vi "CMC_Homework_03_V2.vi"() -> ()   [LabVIEW 2013]
uses:
  <vilib>/gmath/NI_Gmath.lvlib
panel:
  in  "Formulae":string="x*ln(x)*sin(x^2)"
  in  "stop":bool
  out "Middle Bound":dbl
  in  "Lower Bound":dbl
  in  "Upper Bound":dbl
  in  "Tolerance":dbl min=0.0
  out "Calculated Tolerance":dbl
  out "Roots of F(x) found to Tolerance":string[](array[string])
  # "Created in Collaboration with Sarah Bailey & Alex Offredi"
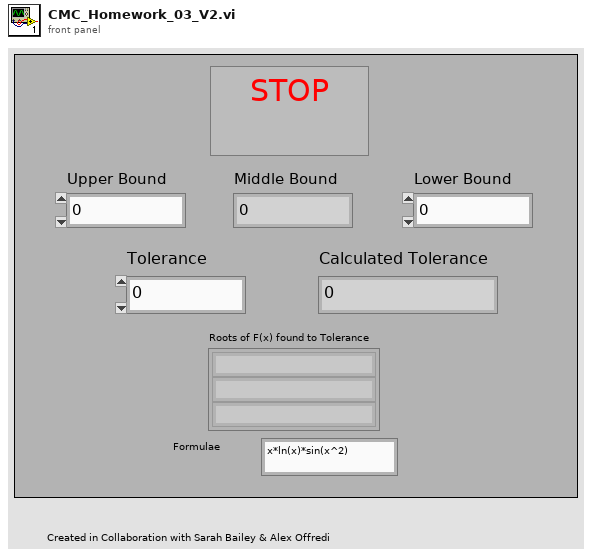
[diagram p1: front panel]
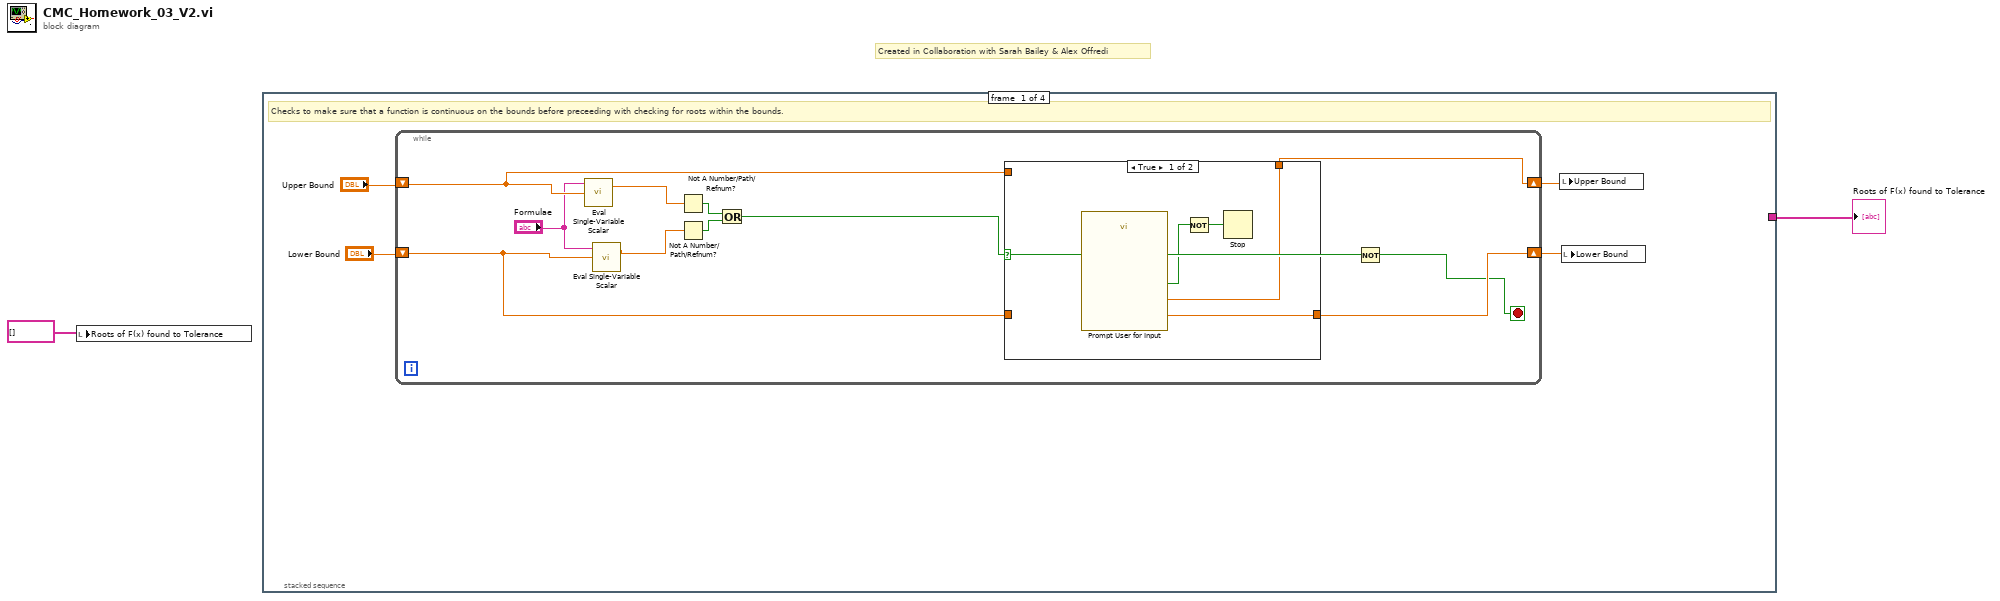
[diagram p0: block diagram]
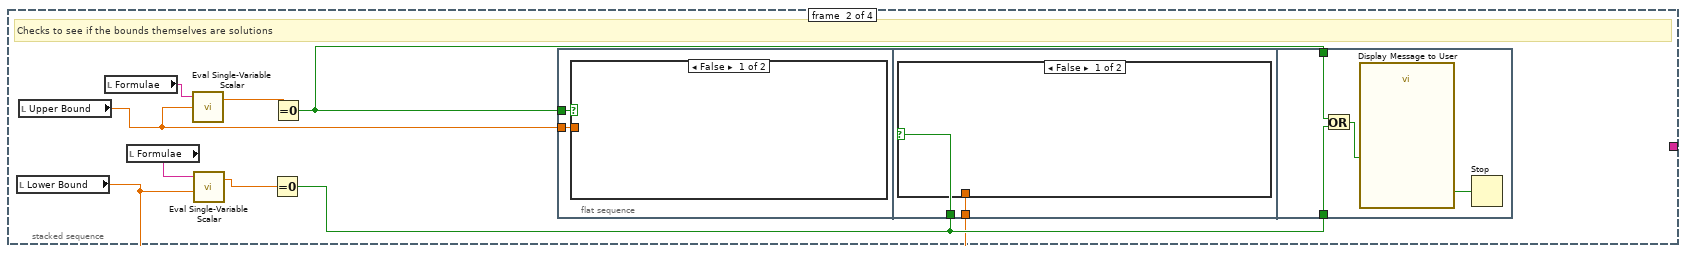
[diagram p3: hidden frame]
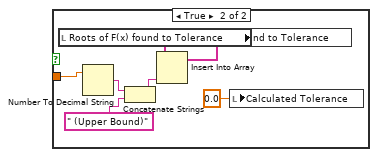
[diagram p4: hidden frame]
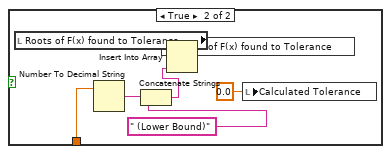
[diagram p5: hidden frame]
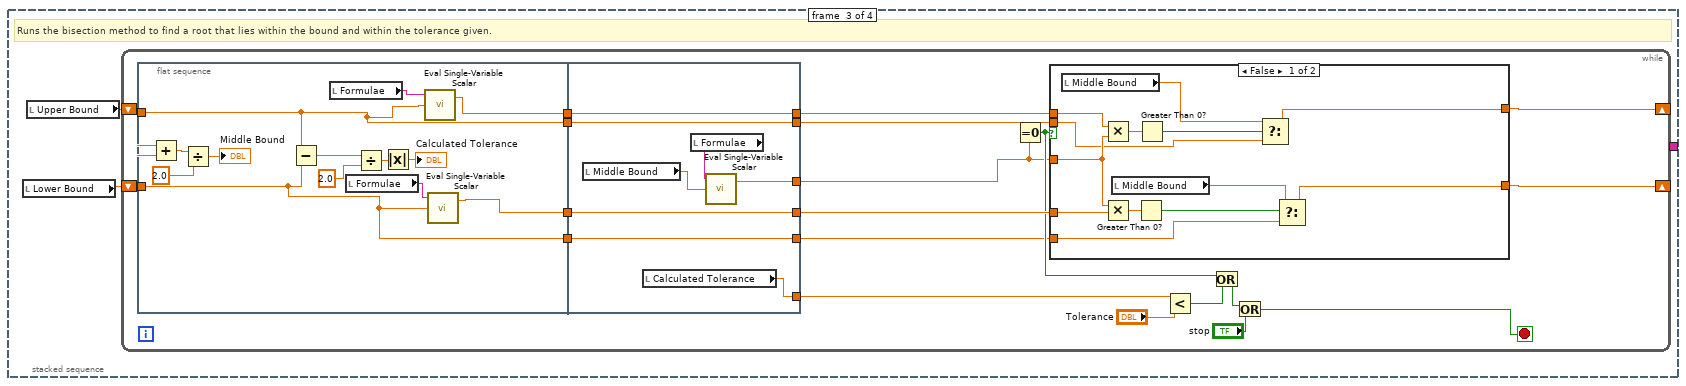
[diagram p6: hidden frame]
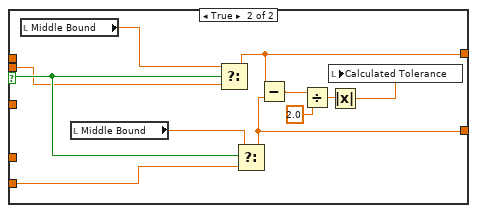
[diagram p7: hidden frame]
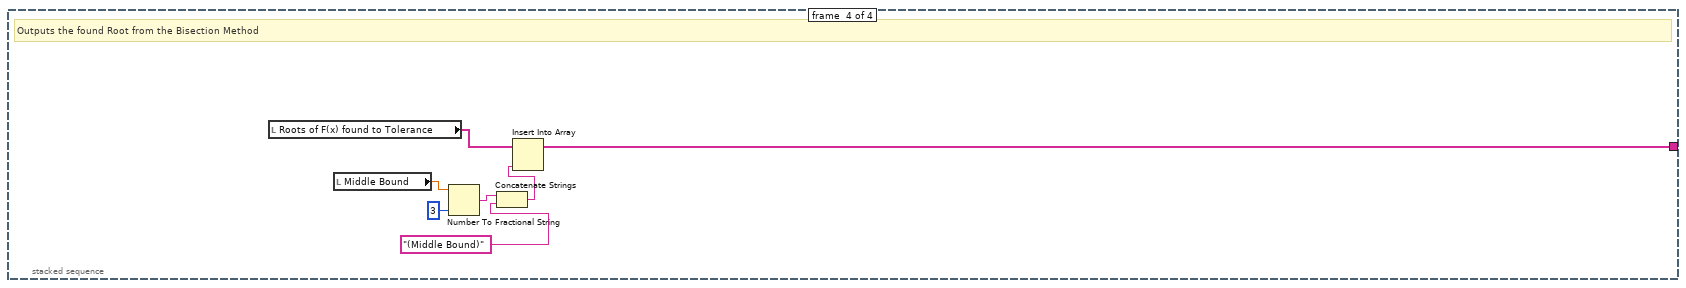
[diagram p8: hidden frame]
diagram:
  # "Created in Collaboration with Sarah Bailey & Alex Offredi"
  n1 = local write "Roots of F(x) found to Tolerance"(string[] [] ("Roots of F(x) found to Tolerance")) -> ()
  n2 = stacked-sequence {
    tunnel: [_ _ _ w122] -> w2
    frame #0 {
      # "Checks to make sure that a function is continuous on the bounds before preceeding with checking for roots within the bounds."
      n3 = while {
        shift-right: [w15] -> w3
        shift-left: "Upper Bound" -> [w11]
        shift-right: [w14] -> w4
        shift-left: "Lower Bound" -> [w9]
        stop <- w12 stop-if-true
        n4 = call <vilib>:"Eval Single-Variable Scalar.vi"("x value"=w11, "formula"="Formulae") -> ("y value"=w7:dbl)  [unwired: 1 in, 1 out]
        n5 = call <vilib>:"Eval Single-Variable Scalar.vi"("x value"=w9, "formula"="Formulae") -> ("y value"=w8:dbl)  [unwired: 1 in, 1 out]
        n6 = Not A Number/Path/Refnum?(number/path/refnum=w7) -> (NaN/Path/Refnum?=w16:bool)
        n7 = Not A Number/Path/Refnum?(number/path/refnum=w8) -> (NaN/Path/Refnum?=w17:bool)
        n8 = Or(x=w16, y=w17) -> (x .or. y?=w13:bool)
        n9 = case shown="True" w13 {
          tunnel: [w19 w22] -> w15
          tunnel: [w18 w23] -> w14
          tunnel: w11 -> [_ w22]
          tunnel: w9 -> [_ w23]
          frame True {
            n10 = call "Prompt User for Input"() -> ("Lower Bound"=w18:dbl, "Upper Bound"=w19:dbl, "OK"=w20:bool)  [unwired: 16 in, 1 out]
            n11 = Not(x=w20) -> (.not. x?=w21:bool)
            n12 = Stop(stop? (T)=w21) -> ()
          }
          frame False {
          }
        }
        n13 = Not(x=w13) -> (.not. x?=w12:bool)
      }
      n14 = local write "Upper Bound"(w3) -> ()
      n15 = local write "Lower Bound"(w4) -> ()
    }
    frame #1 {
      # "Checks to see if the bounds themselves are solutions"
      n16 = local read "Lower Bound"() -> (w25:dbl)
      n17 = local read "Upper Bound"() -> (w28:dbl)
      n18 = local read "Formulae"() -> (w29:string)
      n19 = local read "Formulae"() -> (w26:string)
      n20 = call <vilib>:"Eval Single-Variable Scalar.vi"("x value"=w28, "formula"=w29) -> ("y value"=w27:dbl)  [unwired: 1 in, 1 out]
      n21 = call <vilib>:"Eval Single-Variable Scalar.vi"("x value"=w25, "formula"=w26) -> ("y value"=w24:dbl)  [unwired: 1 in, 1 out]
      n22 = Equal To 0?(x=w24) -> (x = 0?=w31:bool)
      n23 = Equal To 0?(x=w27) -> (x = 0?=w30:bool)
      n24 = flat-sequence {
        tunnel: w30 -> [w33]
        tunnel: w28 -> [w32]
        tunnel: w31 -> [w41]
        tunnel: w25 -> [w42]
        tunnel: w31 -> [w52]
        tunnel: w30 -> [w53]
        frame #0 {
          n25 = case shown="False" w33 {
            tunnel: w32 -> [_ w38]
            frame False {
            }
            frame True {
              n26 = local read "Roots of F(x) found to Tolerance"() -> (w40:string[])
              n27 = Number To Decimal String(number=w38) -> (decimal integer string=w37:string)  [unwired: 1 in]
              n28 = Concatenate Strings(w37, " (Upper Bound)") -> (w35:string)
              n29 = Insert Into Array(array=w40, new element=w35) -> (w39:string[])  [unwired: 1 in]
              n30 = local write "Roots of F(x) found to Tolerance"(w39) -> ()
              n31 = local write "Calculated Tolerance"(0.0 ("Calculated Tolerance")) -> ()
            }
          }
        }
        frame #1 {
          n32 = case shown="False" w41 {
            tunnel: w42 -> [_ w47]
            frame False {
            }
            frame True {
              n33 = local read "Roots of F(x) found to Tolerance"() -> (w49:string[])
              n34 = Number To Decimal String(number=w47) -> (decimal integer string=w46:string)  [unwired: 1 in]
              n35 = Concatenate Strings(w46, " (Lower Bound)") -> (w44:string)
              n36 = Insert Into Array(array=w49, new element=w44) -> (w48:string[])  [unwired: 1 in]
              n37 = local write "Roots of F(x) found to Tolerance"(w48) -> ()
              n38 = local write "Calculated Tolerance"(0.0 ("Calculated Tolerance")) -> ()
            }
          }
        }
        frame #2 {
          n39 = Or(x=w53, y=w52) -> (x .or. y?=w51:bool)
          n40 = call "Display Message to User"("Enable"=w51) -> ("OK"=w50:bool)  [unwired: 9 in, 1 out]
          n41 = Stop(stop? (T)=w50) -> ()
        }
      }
    }
    frame #2 {
      # "Runs the bisection method to find a root that lies within the bound and within the tolerance given."
      n42 = local read "Lower Bound"() -> (w54:dbl)
      n43 = local read "Upper Bound"() -> (w55:dbl)
      n44 = while {
        shift-right: [w71] -> _
        shift-left: w55 -> [w75]
        shift-right: [w70] -> _
        shift-left: w54 -> [w74]
        stop <- w68 stop-if-true
        n45 = flat-sequence {
          tunnel: w75 -> [w105]
          tunnel: w74 -> [w102]
          tunnel: [w104] -> w61
          tunnel: [w103] -> w60
          tunnel: [w105] -> w59
          tunnel: [w102] -> w58
          tunnel: [w117] -> w62
          tunnel: [w118] -> w63
          tunnel: [w119] -> w72
          tunnel: [w120] -> w73
          tunnel: w61 -> [w120]
          tunnel: w60 -> [w119]
          tunnel: w59 -> [w118]
          tunnel: w58 -> [w117]
          tunnel: [w114] -> w57
          tunnel: [w113] -> w56
          frame #0 {
            n46 = Add(x=w105, y=w102) -> (x+y=w111:dbl)
            n47 = Divide(x=w111, y=2.0) -> (x/y=→"Middle Bound":dbl)
            n48 = Subtract(x=w105, y=w102) -> (x-y=w109:dbl)
            n49 = local read "Formulae"() -> (w101:string)
            n50 = local read "Formulae"() -> (w100:string)
            n51 = Divide(x=w109, y=2.0) -> (x/y=w107:dbl)
            n52 = Absolute Value(x=w107) -> (abs(x)=→"Calculated Tolerance":dbl)
            n53 = call <vilib>:"Eval Single-Variable Scalar.vi"("x value"=w105, "formula"=w101) -> ("y value"=w104:dbl)  [unwired: 1 in, 1 out]
            n54 = call <vilib>:"Eval Single-Variable Scalar.vi"("x value"=w102, "formula"=w100) -> ("y value"=w103:dbl)  [unwired: 1 in, 1 out]
          }
          frame #1 {
            n55 = local read "Middle Bound"() -> (w116:dbl)
            n56 = local read "Calculated Tolerance"() -> (w113:dbl)
            n57 = local read "Formulae"() -> (w115:string)
            n58 = call <vilib>:"Eval Single-Variable Scalar.vi"("x value"=w116, "formula"=w115) -> ("y value"=w114:dbl)  [unwired: 1 in, 1 out]
          }
        }
        n59 = Equal To 0?(x=w57) -> (x = 0?=w66:bool)
        n60 = case shown="False" w66 {
          selector: w66 -> [_ w91]
          tunnel: w73 -> [w78 _]
          tunnel: w72 -> [w80 _]
          tunnel: [w85 w95] -> w71
          tunnel: w57 -> [w79 _]
          tunnel: [w82 w94] -> w70
          tunnel: w63 -> [w77 w89]
          tunnel: w62 -> [w76 w90]
          frame False {
            n61 = local read "Middle Bound"() -> (w81:dbl)
            n62 = Multiply(x=w78, y=w79) -> (x*y=w88:dbl)
            n63 = Multiply(x=w79, y=w80) -> (x*y=w87:dbl)
            n64 = local read "Middle Bound"() -> (w83:dbl)
            n65 = Greater Than 0?(x=w87) -> (x > 0?=w84:bool)
            n66 = Greater Than 0?(x=w88) -> (x > 0?=w86:bool)
            n67 = Select(t=w81, s=w86, f=w77) -> (s? t:f=w85:dbl)
            n68 = Select(t=w83, s=w84, f=w76) -> (s? t:f=w82:dbl)
          }
          frame True {
            n69 = local read "Middle Bound"() -> (w98:dbl)
            n70 = local read "Middle Bound"() -> (w99:dbl)
            n71 = Select(t=w98, s=w91, f=w89) -> (s? t:f=w95:dbl)
            n72 = Select(t=w99, s=w91, f=w90) -> (s? t:f=w94:dbl)
            n73 = Subtract(x=w95, y=w94) -> (x-y=w96:dbl)
            n74 = Divide(x=w96, y=2.0) -> (x/y=w93:dbl)
            n75 = Absolute Value(x=w93) -> (abs(x)=w92:dbl)
            n76 = local write "Calculated Tolerance"(w92) -> ()
          }
        }
        n77 = Less?(x=w56, y="Tolerance") -> (x < y?=w65:bool)
        n78 = Or(x=w66, y=w65) -> (x .or. y?=w64:bool)
        n79 = Or(x=w64, y="stop") -> (x .or. y?=w68:bool)
      }
    }
    frame #3 {
      # "Outputs the found Root from the Bisection Method"
      n80 = local read "Roots of F(x) found to Tolerance"() -> (w127:string[])
      n81 = local read "Middle Bound"() -> (w126:dbl)
      n82 = Number To Fractional String(number=w126, precision (6)=i16 3) -> (F-format string=w125:string)  [unwired: 2 in]
      n83 = Concatenate Strings(w125, "(Middle Bound)") -> (w123:string)
      n84 = Insert Into Array(array=w127, new element=w123) -> (w122:string[])  [unwired: 1 in]
    }
  }
  "Roots of F(x) found to Tolerance" <- w2
